vi "PwF_ToF_Open.vi"(6 "Tsamp_ms":u16=50, 8 "error in":errorcluster, 9 "Ranging Mode":T1, 10 "Device ID":u8) -> (0 "error out":errorcluster, 3 "PwF ToF Ref":T2)   [LabVIEW 2018]
uses:
  ToF_TypeDef/PwF ToF Ref.ctl
  ToF_TypeDef/PwF ToF RangingMode.ctl
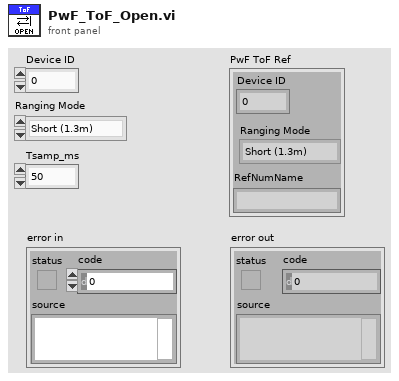
[diagram p1: front panel]
types:
  T1 = typedef "PwF ToF RangingMode.ctl" = enum8{"Short (1.3m)", "Medium (2m)", "Long (4m)"}
  T2 = typedef "PwF ToF Ref.ctl" = cluster{"Device ID":u8, "Ranging Mode":T1, "RefNumName":string}
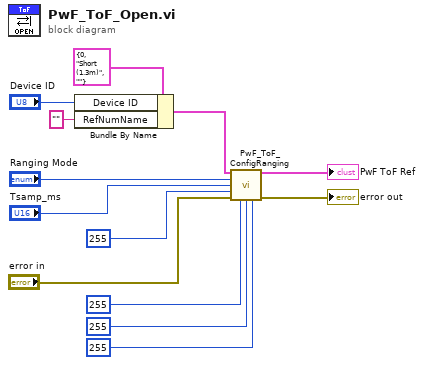
[diagram p0: block diagram]
diagram:
  n1 = Bundle By Name(cluster=T2 {"Device ID"=0, "Ranging Mode"=enum."Short (1.3m)", "RefNumName"=""} ("type"), "Device ID"="Device ID", "RefNumName"="") -> (w8:T2)
  n2 = call "PwF_ToF_ConfigRanging.vi"("PwF ToF Ref"=w8, "Ranging Mode"="Ranging Mode", "Tsamp_ms"="Tsamp_ms", "ROI_TL_Xcoord"=u8 255, "error in (no error)"="error in", "ROI_TL_Ycoord"=u8 255, "ROI_BR_Xcoord"=u8 255, "ROI_BR_Ycoord"=u8 255) -> ("PwF ToF Ref"=→"PwF ToF Ref":T2, "error out"=→"error out":errorcluster)  [unwired: 6 in]
